vi "Bundle and Sort.vi"(1 "Data":dbl[](array[numeric]), 2 "Frequency":dbl[](array[numeric]), 3 "Time":dbl[](array[numeric])) -> (8 "Bundled Array":T1(array[cluster]))   [LabVIEW 2014, in "Melody Extraction.lvlib"]
uses:
  Melody Extraction.lvlib
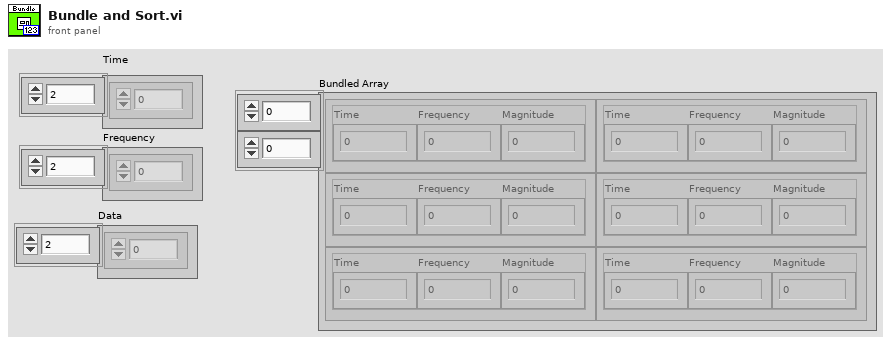
[diagram p1: front panel]
types:
  T1 = cluster{"Time":dbl, "Frequency":dbl, "Magnitude":dbl}[][]
  T2 = cluster{"Numeric Control":dbl, "Numeric Control":dbl, "Numeric Control":dbl}[]
  T3 = cluster{"Numeric Control":dbl, "Numeric Control":dbl, "Numeric Control":dbl}
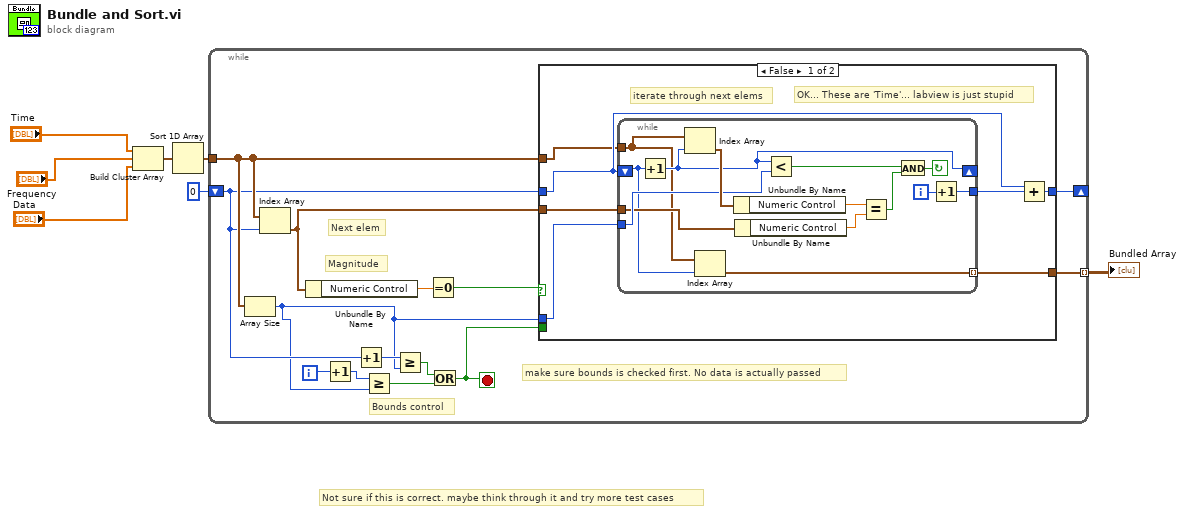
[diagram p0: block diagram]
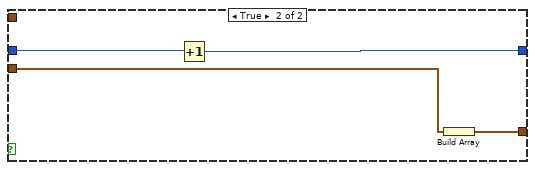
[diagram p2: hidden frame]
diagram:
  # "Not sure if this is correct. maybe think through it and try more test cases"
  n1 = Build Cluster Array("Time", "Frequency", "Data") -> (w7:T2)
  n2 = Sort 1D Array(array=w7) -> (sorted array=w3:T2)
  n3 = while {
    tunnel: w3 -> [w17]
    shift-right: [w19] -> _
    shift-left: 0 -> [w12]
    tunnel: [w18] -> w2 mode=indexing
    i -> [w11]
    stop <- w9 stop-if-true
    # "make sure bounds is checked first. No data is actually passed"
    # "Next elem"
    # "Bounds control"
    # "Magnitude"
    n4 = Array Size(array=w17) -> (size(s)=w8:i32)
    n5 = Index Array(array=w17, index=w12) -> (element=w20:T3)
    n6 = Unbundle By Name(w20) -> ("Numeric Control"=w21:dbl)
    n7 = Increment(x=w11) -> (x+1=w13:i32)
    n8 = Increment(x=w12) -> (x+1=w15:i32)
    n9 = Greater Or Equal?(x=w13, y=w8) -> (x >= y?=w14:bool)
    n10 = Greater Or Equal?(x=w15, y=w8) -> (x >= y?=w16:bool)
    n11 = Equal To 0?(x=w21) -> (x = 0?=w10:bool)
    n12 = Or(x=w16, y=w14) -> (x .or. y?=w9:bool)
    n13 = case shown="False" w10 {
      tunnel: [w27 w45] -> w19
      tunnel: w12 -> [w26 w46]
      tunnel: w17 -> [w25 _]
      tunnel: [w24 w43] -> w18
      tunnel: w20 -> [w23 w44]
      tunnel: w8 -> [w22 _]
      tunnel: w9 -> [_ _]
      frame False {
        # "iterate through next elems"
        # "OK... These are 'Time'... labview is just stupid"
        n14 = while {
          tunnel: [w39] -> w28
          tunnel: w23 -> [w32]
          tunnel: w25 -> [w30]
          shift-right: [w35] -> _
          shift-left: w26 -> [w31]
          tunnel: w22 -> [w34]
          tunnel: [w29] -> w24 mode=indexing
          i -> [w40]
          stop <- w37 continue-if-true
          n15 = Increment(x=w31) -> (x+1=w35:i32)
          n16 = Index Array(array=w30, index=w35) -> (element=w38:T3)
          n17 = Index Array(array=w30, index=w31) -> (element=w29:T3)
          n18 = Unbundle By Name(w38) -> ("Numeric Control"=w42:dbl)
          n19 = Unbundle By Name(w32) -> ("Numeric Control"=w41:dbl)
          n20 = Less?(x=w35, y=w34) -> (x < y?=w33:bool)
          n21 = Equal?(x=w42, y=w41) -> (x = y?=w36:bool)
          n22 = And(x=w33, y=w36) -> (x .and. y?=w37:bool)
          n23 = Increment(x=w40) -> (x+1=w39:i32)
        }
        n24 = Add(x=w26, y=w28) -> (x+y=w27:i32)
      }
      frame True {
        n25 = Increment(x=w46) -> (x+1=w45:i32)
        n26 = Build Array(w44) -> (w43:T2)
      }
    }
  }
  "Bundled Array" <- w2
